vi "Prepare_dataST.vi"(1 "Active Sensors":bool[](array[boolean]), 2 "ranges":bool[](array[boolean]), 3 "Controls[]":refnum<vi>[](array[refnum]), 4 "Flag_215":bool, 5 "error in":errorcluster, 6 "struct":bool, 7 "chkeach_ch":bool) -> (12 "Meas_rang":i32[](array[numeric]), 13 "Refdata_struct":refnum<k24>[](array[refnum]), 15 "Meas_monitor_struct":refnum<k24>[](array[refnum]), 16 "Data_struct":refnum<k24>[](array[refnum]), 17 "Ref_monitordata_struct":refnum<k24>[](array[refnum]), 18 "Mergedata_struct":refnum<k24>[](array[refnum]), 19 "error out":errorcluster)   [LabVIEW 2017]
doc: "prepare data struct & hold instrument condition"
uses:
  D:/test/ILSTS/LV_IL/LV_IL_Sample_x64/DLL/STSProcess.dll
  DLL/STSProcess.dll
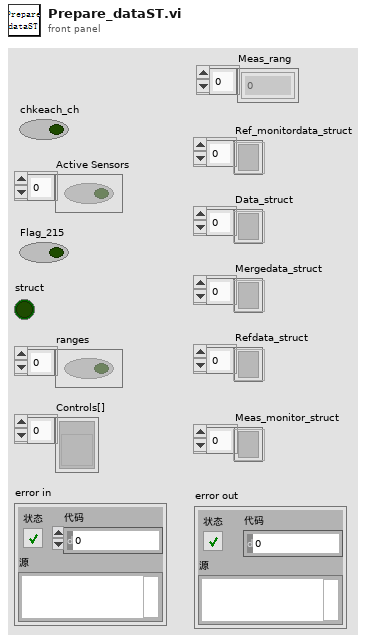
[diagram p1: front panel]
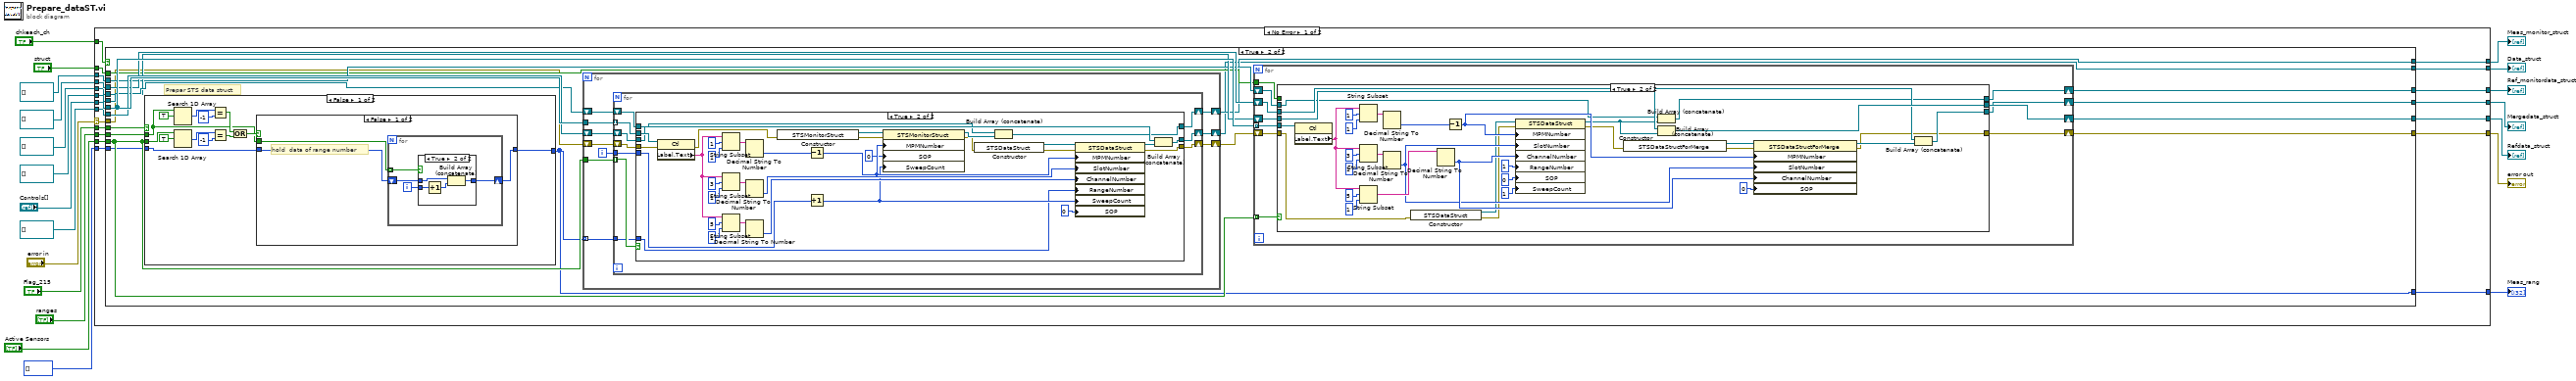
[diagram p0: block diagram]
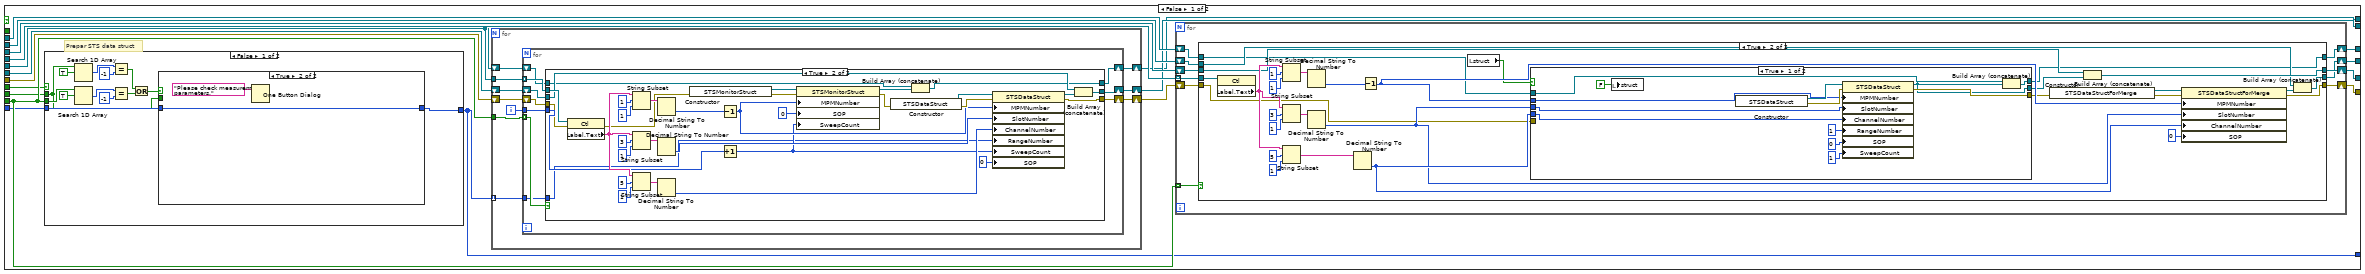
[diagram p2: hidden frame]
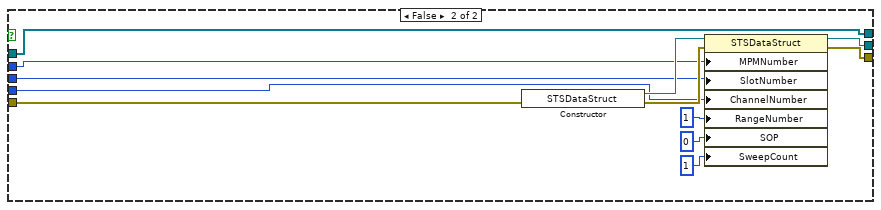
[diagram p4: hidden frame]
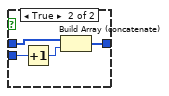
[diagram p7: hidden frame]
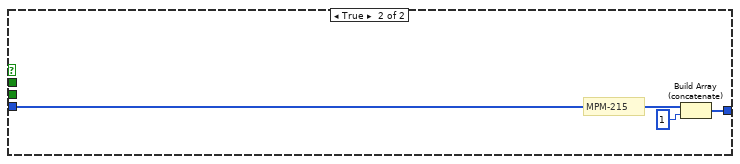
[diagram p8: hidden frame]
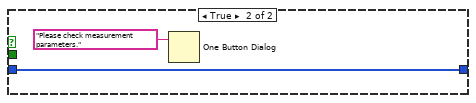
[diagram p12: hidden frame]
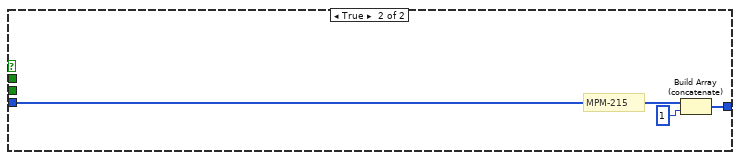
[diagram p13: hidden frame]
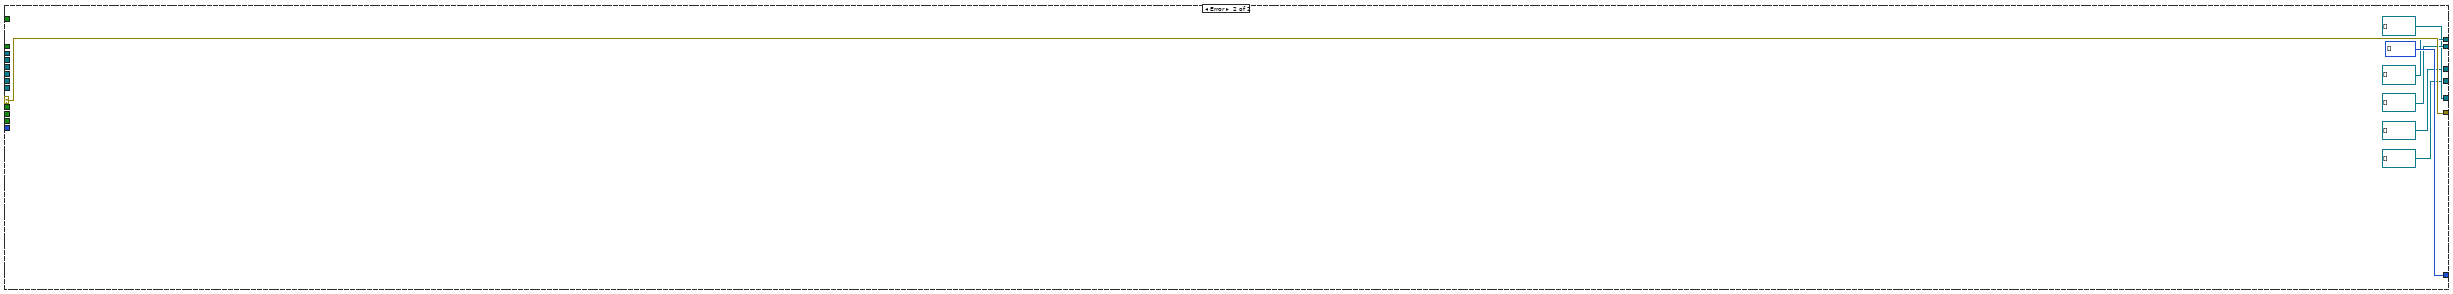
[diagram p14: hidden frame]
diagram:
  n1 = case shown="No Error" "error in" {
    selector: "error in" -> [w21 w378]
    tunnel: "ranges" -> [w40 _]
    tunnel: "Flag_215" -> [w39 _]
    tunnel: "Controls[]" -> [w38 _]
    tunnel: "Active Sensors" -> [w37 _]
    tunnel: "chkeach_ch" -> [w36 _]
    tunnel: "struct" -> [w35 _]
    tunnel: refnum<k24>[] [] ("Data_struct") -> [w34 _]
    tunnel: refnum<k24>[] [] ("Ref_monitordata_struct") -> [w33 _]
    tunnel: refnum<k24>[] [] ("Mergedata_struct") -> [w32 _]
    tunnel: refnum<k24>[] [] ("Meas_monitor_struct") -> [w31 _]
    tunnel: refnum<k24>[] [] ("Refdata_struct") -> [w30 _]
    tunnel: [w29 refnum<k24>[] [] ("Mergedata_struct")] -> w9
    tunnel: [w28 refnum<k24>[] [] ("Data_struct")] -> w8
    tunnel: [w27 refnum<k24>[] [] ("Meas_monitor_struct")] -> w7
    tunnel: [w26 refnum<k24>[] [] ("Refdata_struct")] -> w6
    tunnel: [w25 refnum<k24>[] [] ("Ref_monitordata_struct")] -> w5
    tunnel: i32[] [] ("Meas_rang") -> [w24 _]
    tunnel: [w23 i32[] [] ("Meas_rang")] -> w3
    tunnel: [w22 w378] -> w1
    frame No Error {
      n2 = case shown="True" w36 {
        tunnel: w37 -> [w58 w234]
        tunnel: w38 -> [w59 w235]
        tunnel: w34 -> [w57 w233]
        tunnel: w31 -> [w56 w232]
        tunnel: w30 -> [w55 w231]
        tunnel: w32 -> [w54 w230]
        tunnel: w33 -> [w53 w229]
        tunnel: w24 -> [w52 w228]
        tunnel: w39 -> [w51 w227]
        tunnel: w40 -> [w50 w226]
        tunnel: w35 -> [_ w225]
        tunnel: [w49 w222] -> w29
        tunnel: [w48 w223] -> w28
        tunnel: [w47 w224] -> w27
        tunnel: [w46 w220] -> w26
        tunnel: [w45 w221] -> w25
        tunnel: [w44 w219] -> w23
        tunnel: [w41 w218] -> w22
        tunnel: w21 -> [w42 w216]
        frame False {
          # "Prepar STS data struct"
          n3 = case shown="False" w51 {
            tunnel: w52 -> [w188 w215]
            tunnel: [w187 w213] -> w44
            tunnel: w58 -> [w198 _]
            tunnel: w50 -> [w186 _]
            frame False {
              n4 = Search 1D Array(1D array=w186, element=TRUE ("元素")) -> (index of element=w193:i32)  [unwired: 1 in]
              n5 = Search 1D Array(1D array=w198, element=TRUE ("元素")) -> (index of element=w196:i32)  [unwired: 1 in]
              n6 = Equal?(x=w193, y=-1) -> (x = y?=w191:bool)
              n7 = Equal?(x=w196, y=-1) -> (x = y?=w190:bool)
              n8 = Or(x=w191, y=w190) -> (x .or. y?=w189:bool)
              n9 = case shown="True" w189 {
                tunnel: w186 -> [w201 _]
                tunnel: w188 -> [w200 w211]
                tunnel: [w199 w211] -> w187
                frame False {
                  # "hold  data of range number"
                  n10 = for {
                    tunnel: w201 -> [w205] mode=indexing
                    shift-right: [w202] -> w199
                    shift-left: w200 -> [w204]
                    i -> [w203]
                    n11 = case shown="False" w205 {
                      tunnel: w204 -> [w206 w210]
                      tunnel: w203 -> [_ w208]
                      tunnel: [w206 w207] -> w202
                      frame False {
                      }
                      frame True {
                        n12 = Increment(x=w208) -> (x+1=w209:i32)
                        n13 = Build Array (concatenate)(w210, w209) -> (w207:i32[])
                      }
                    }
                  }
                }
                frame True {
                  n14 = One Button Dialog(message="Please check measurement parameters." ("消息")) -> ()  [unwired: 1 in, 1 out]
                }
              }
            }
            frame True {
              # "MPM-215"
              n15 = Build Array (concatenate)(w215, 1) -> (w213:i32[])
            }
          }
          n16 = for {
            tunnel: w58 -> [w138]
            tunnel: w59 -> [w137]
            tunnel: w44 -> [w136] mode=indexing
            shift-right: [w134] -> w48
            shift-left: w57 -> [w135]
            shift-right: [w131] -> w47
            shift-left: w56 -> [w132]
            shift-right: [w130] -> w43
            shift-left: w42 -> [w129]
            i -> [w133]
            n17 = for {
              tunnel: w138 -> [w148] mode=indexing
              tunnel: w137 -> [w147] mode=indexing
              tunnel: w136 -> [w139]
              shift-right: [w145] -> w134
              shift-left: w135 -> [w146]
              tunnel: w133 -> [w144]
              shift-right: [w142] -> w131
              shift-left: w132 -> [w143]
              shift-right: [w141] -> w130
              shift-left: w129 -> [w140]
              n18 = case shown="True" w148 {
                tunnel: w147 -> [_ w185]
                tunnel: w146 -> [w151 w171]
                tunnel: [w151 w169] -> w145
                tunnel: w144 -> [_ w166]
                tunnel: w143 -> [w150 w159]
                tunnel: [w150 w157] -> w142
                tunnel: [w149 w154] -> w141
                tunnel: w140 -> [w149 w153]
                tunnel: w139 -> [_ w152]
                frame False {
                }
                frame True {
                  n19 = property class="Ctl"(reference=w185, error in=w153) -> (error out=w156:errorcluster, "Label.Text"=w180:string)  [unwired: 1 out]
                  n20 = String Subset(string=w180, offset (0)=1 ("偏移量(0)"), length (rest)=1 ("长度（剩余）")) -> (substring=w176:string)
                  n21 = String Subset(string=w180, offset (0)=3 ("偏移量(0)"), length (rest)=1 ("长度（剩余）")) -> (substring=w177:string)
                  n22 = String Subset(string=w180, offset (0)=5 ("偏移量(0)"), length (rest)=1 ("长度（剩余）")) -> (substring=w175:string)
                  n23 = Decimal String To Number(string=w176) -> (number=w174:i32)  [unwired: 2 in, 1 out]
                  n24 = Decimal String To Number(string=w177) -> (number=w168:i32)  [unwired: 2 in, 1 out]
                  n25 = Decimal String To Number(string=w175) -> (number=w167:i32)  [unwired: 2 in, 1 out]
                  n26 = constructor class="STSMonitorStruct"(error in=w156) -> (reference out=w163:refnum<k24>, error out=w164:errorcluster)  [unwired: 2 in, 1 out]
                  n27 = Decrement(x=w174) -> (x-1=w162:i32)
                  n28 = Increment(x=w166) -> (x+1=w160:i32)
                  n29 = property class="STSMonitorStruct"(reference=w163, error in=w164, "MPMNumber"=w162, "SOP"=0, "SweepCount"=w160) -> (reference out=w158:refnum<k24>, error out=w155:errorcluster)
                  n30 = constructor class="STSDataStruct"(error in=w155) -> (reference out=w173:refnum<k24>, error out=w172:errorcluster)  [unwired: 2 in, 1 out]
                  n31 = Build Array (concatenate)(w159, w158) -> (w157:refnum<k24>[])
                  n32 = property on="属性节点" class="STSDataStruct"(reference=w173, error in=w172, "MPMNumber"=w162, "SlotNumber"=w168, "ChannelNumber"=w167, "RangeNumber"=w152, "SweepCount"=w160, "SOP"=0) -> (reference out=w170:refnum<k24>, error out=w154:errorcluster)
                  n33 = Build Array (concatenate)(w171, w170) -> (w169:refnum<k24>[])
                }
              }
            }
          }
          n34 = for {
            tunnel: w59 -> [w68] mode=indexing
            tunnel: w58 -> [w69] mode=indexing
            shift-right: [w66] -> w46
            shift-left: w55 -> [w67]
            shift-right: [w64] -> w49
            shift-left: w54 -> [w65]
            shift-right: [w62] -> w45
            shift-left: w53 -> [w63]
            shift-right: [w60] -> w41
            shift-left: w43 -> [w61]
            n35 = case shown="True" w69 {
              tunnel: w68 -> [_ w93]
              tunnel: w67 -> [w72 w84]
              tunnel: [w72 w82] -> w66
              tunnel: w65 -> [w73 w81]
              tunnel: [w73 w79] -> w64
              tunnel: w63 -> [w71 w78]
              tunnel: [w71 w77] -> w62
              tunnel: w61 -> [w70 w76]
              tunnel: [w70 w75] -> w60
              frame False {
              }
              frame True {
                n36 = property class="Ctl"(reference=w93) -> ("Label.Text"=w92:string)  [unwired: 1 in, 2 out]
                n37 = String Subset(string=w92, offset (0)=1 ("偏移量(0)"), length (rest)=1 ("长度（剩余）")) -> (substring=w96:string)
                n38 = String Subset(string=w92, offset (0)=3 ("偏移量(0)"), length (rest)=1 ("长度（剩余）")) -> (substring=w97:string)
                n39 = String Subset(string=w92, offset (0)=5 ("偏移量(0)"), length (rest)=1 ("长度（剩余）")) -> (substring=w95:string)
                n40 = Decimal String To Number(string=w96) -> (number=w94:i32)  [unwired: 2 in, 1 out]
                n41 = Decimal String To Number(string=w97) -> (number=w87:i32)  [unwired: 2 in, 1 out]
                n42 = Decimal String To Number(string=w95) -> (number=w88:i32)  [unwired: 2 in, 1 out]
                n43 = Decrement(x=w94) -> (x-1=w86:i32)
                n44 = local read "struct"() -> (w74:bool)
                n45 = case shown="True" w74 {
                  tunnel: w88 -> [w111 w123]
                  tunnel: w87 -> [w110 w122]
                  tunnel: w86 -> [w109 w121]
                  tunnel: [w108 w120] -> w85
                  tunnel: [w106 w119] -> w83
                  tunnel: w78 -> [w107 w118]
                  tunnel: [w105 w118] -> w77
                  tunnel: w76 -> [_ w117]
                  frame True {
                    n46 = local write "struct"(FALSE ("struct")) -> ()
                    n47 = constructor class="STSDataStruct"() -> (reference out=w115:refnum<k24>, error out=w116:errorcluster)  [unwired: 3 in, 1 out]
                    n48 = property class="STSDataStruct"(reference=w115, error in=w116, "MPMNumber"=w109, "SlotNumber"=w110, "ChannelNumber"=w111, "RangeNumber"=1, "SOP"=0, "SweepCount"=1) -> (reference out=w106:refnum<k24>, error out=w108:errorcluster)
                    n49 = Build Array (concatenate)(w107, w106) -> (w105:refnum<k24>[])
                  }
                  frame False {
                    n50 = constructor class="STSDataStruct"(error in=w117) -> (reference out=w127:refnum<k24>, error out=w128:errorcluster)  [unwired: 2 in, 1 out]
                    n51 = property class="STSDataStruct"(reference=w127, error in=w128, "MPMNumber"=w121, "SlotNumber"=w122, "ChannelNumber"=w123, "RangeNumber"=1, "SOP"=0, "SweepCount"=1) -> (reference out=w119:refnum<k24>, error out=w120:errorcluster)
                  }
                }
                n52 = constructor class="STSDataStructForMerge"(error in=w85) -> (reference out=w91:refnum<k24>, error out=w90:errorcluster)  [unwired: 2 in, 1 out]
                n53 = Build Array (concatenate)(w84, w83) -> (w82:refnum<k24>[])
                n54 = property class="STSDataStructForMerge"(reference=w91, error in=w90, "MPMNumber"=w86, "SlotNumber"=w87, "ChannelNumber"=w88, "SOP"=0) -> (reference out=w80:refnum<k24>, error out=w75:errorcluster)
                n55 = Build Array (concatenate)(w81, w80) -> (w79:refnum<k24>[])
              }
            }
          }
        }
        frame True {
          # "Prepar STS data struct"
          n56 = case shown="False" w227 {
            tunnel: w228 -> [w344 w371]
            tunnel: [w343 w369] -> w219
            tunnel: w234 -> [w354 _]
            tunnel: w226 -> [w342 _]
            frame False {
              n57 = Search 1D Array(1D array=w342, element=TRUE ("元素")) -> (index of element=w349:i32)  [unwired: 1 in]
              n58 = Search 1D Array(1D array=w354, element=TRUE ("元素")) -> (index of element=w352:i32)  [unwired: 1 in]
              n59 = Equal?(x=w349, y=-1) -> (x = y?=w347:bool)
              n60 = Equal?(x=w352, y=-1) -> (x = y?=w346:bool)
              n61 = Or(x=w347, y=w346) -> (x .or. y?=w345:bool)
              n62 = case shown="False" w345 {
                tunnel: w342 -> [w357 _]
                tunnel: w344 -> [w356 w367]
                tunnel: [w355 w367] -> w343
                frame False {
                  # "hold  data of range number"
                  n63 = for {
                    tunnel: w357 -> [w361] mode=indexing
                    shift-right: [w358] -> w355
                    shift-left: w356 -> [w360]
                    i -> [w359]
                    n64 = case shown="True" w361 {
                      tunnel: w360 -> [w362 w366]
                      tunnel: w359 -> [_ w364]
                      tunnel: [w362 w363] -> w358
                      frame False {
                      }
                      frame True {
                        n65 = Increment(x=w364) -> (x+1=w365:i32)
                        n66 = Build Array (concatenate)(w366, w365) -> (w363:i32[])
                      }
                    }
                  }
                }
                frame True {
                  n67 = One Button Dialog(message="Please check measurement parameters." ("消息")) -> ()  [unwired: 1 in, 1 out]
                }
              }
            }
            frame True {
              # "MPM-215"
              n68 = Build Array (concatenate)(w371, 1) -> (w369:i32[])
            }
          }
          n69 = for {
            tunnel: w234 -> [w294]
            tunnel: w235 -> [w293]
            tunnel: w219 -> [w292] mode=indexing
            shift-right: [w290] -> w223
            shift-left: w233 -> [w291]
            shift-right: [w287] -> w224
            shift-left: w232 -> [w288]
            shift-right: [w286] -> w217
            shift-left: w216 -> [w285]
            i -> [w289]
            n70 = for {
              tunnel: w294 -> [w304] mode=indexing
              tunnel: w293 -> [w303] mode=indexing
              tunnel: w292 -> [w295]
              shift-right: [w301] -> w290
              shift-left: w291 -> [w302]
              tunnel: w289 -> [w300]
              shift-right: [w298] -> w287
              shift-left: w288 -> [w299]
              shift-right: [w297] -> w286
              shift-left: w285 -> [w296]
              n71 = case shown="True" w304 {
                tunnel: w303 -> [_ w341]
                tunnel: w302 -> [w307 w327]
                tunnel: [w307 w325] -> w301
                tunnel: w300 -> [_ w322]
                tunnel: w299 -> [w306 w315]
                tunnel: [w306 w313] -> w298
                tunnel: [w305 w310] -> w297
                tunnel: w296 -> [w305 w309]
                tunnel: w295 -> [_ w308]
                frame False {
                }
                frame True {
                  n72 = property class="Ctl"(reference=w341, error in=w309) -> (error out=w311:errorcluster, "Label.Text"=w336:string)  [unwired: 1 out]
                  n73 = String Subset(string=w336, offset (0)=1 ("偏移量(0)"), length (rest)=1 ("长度（剩余）")) -> (substring=w332:string)
                  n74 = String Subset(string=w336, offset (0)=3 ("偏移量(0)"), length (rest)=1 ("长度（剩余）")) -> (substring=w333:string)
                  n75 = String Subset(string=w336, offset (0)=5 ("偏移量(0)"), length (rest)=1 ("长度（剩余）")) -> (substring=w331:string)
                  n76 = Decimal String To Number(string=w332) -> (number=w330:i32)  [unwired: 2 in, 1 out]
                  n77 = Decimal String To Number(string=w333) -> (number=w324:i32)  [unwired: 2 in, 1 out]
                  n78 = Decimal String To Number(string=w331) -> (number=w323:i32)  [unwired: 2 in, 1 out]
                  n79 = constructor class="STSMonitorStruct"(error in=w311) -> (reference out=w319:refnum<k24>, error out=w320:errorcluster)  [unwired: 2 in, 1 out]
                  n80 = Decrement(x=w330) -> (x-1=w318:i32)
                  n81 = Increment(x=w322) -> (x+1=w316:i32)
                  n82 = property class="STSMonitorStruct"(reference=w319, error in=w320, "MPMNumber"=w318, "SOP"=0, "SweepCount"=w316) -> (reference out=w314:refnum<k24>, error out=w312:errorcluster)
                  n83 = constructor class="STSDataStruct"(error in=w312) -> (reference out=w329:refnum<k24>, error out=w328:errorcluster)  [unwired: 2 in, 1 out]
                  n84 = Build Array (concatenate)(w315, w314) -> (w313:refnum<k24>[])
                  n85 = property on="属性节点" class="STSDataStruct"(reference=w329, error in=w328, "MPMNumber"=w318, "SlotNumber"=w324, "ChannelNumber"=w323, "RangeNumber"=w308, "SweepCount"=w316, "SOP"=0) -> (reference out=w326:refnum<k24>, error out=w310:errorcluster)
                  n86 = Build Array (concatenate)(w327, w326) -> (w325:refnum<k24>[])
                }
              }
            }
          }
          n87 = for {
            tunnel: w235 -> [w245] mode=indexing
            tunnel: w234 -> [w246] mode=indexing
            shift-right: [w243] -> w220
            shift-left: w231 -> [w244]
            shift-right: [w241] -> w222
            shift-left: w230 -> [w242]
            shift-right: [w239] -> w221
            shift-left: w229 -> [w240]
            tunnel: w225 -> [w238]
            shift-right: [w237] -> w218
            shift-left: w217 -> [w236]
            n88 = case shown="True" w246 {
              tunnel: w245 -> [_ w274]
              tunnel: w244 -> [w249 w265]
              tunnel: [w249 w263] -> w243
              tunnel: w242 -> [w250 w262]
              tunnel: [w250 w260] -> w241
              tunnel: w240 -> [w248 w259]
              tunnel: [w248 w258] -> w239
              tunnel: w238 -> [_ _]
              tunnel: [w247 w257] -> w237
              tunnel: w236 -> [w247 w251]
              frame False {
              }
              frame True {
                n89 = property class="Ctl"(reference=w274) -> ("Label.Text"=w273:string)  [unwired: 1 in, 2 out]
                n90 = String Subset(string=w273, offset (0)=1 ("偏移量(0)"), length (rest)=1 ("长度（剩余）")) -> (substring=w277:string)
                n91 = String Subset(string=w273, offset (0)=3 ("偏移量(0)"), length (rest)=1 ("长度（剩余）")) -> (substring=w278:string)
                n92 = String Subset(string=w273, offset (0)=5 ("偏移量(0)"), length (rest)=1 ("长度（剩余）")) -> (substring=w276:string)
                n93 = Decimal String To Number(string=w277) -> (number=w275:i32)  [unwired: 2 in, 1 out]
                n94 = Decimal String To Number(string=w278) -> (number=w268:i32)  [unwired: 2 in, 1 out]
                n95 = constructor class="STSDataStruct"(error in=w251) -> (reference out=w255:refnum<k24>, error out=w256:errorcluster)  [unwired: 2 in, 1 out]
                n96 = Decimal String To Number(string=w276) -> (number=w269:i32)  [unwired: 2 in, 1 out]
                n97 = Decrement(x=w275) -> (x-1=w267:i32)
                n98 = property class="STSDataStruct"(reference=w255, error in=w256, "MPMNumber"=w267, "SlotNumber"=w268, "ChannelNumber"=w269, "RangeNumber"=1, "SOP"=0, "SweepCount"=1) -> (reference out=w264:refnum<k24>, error out=w266:errorcluster)
                n99 = constructor class="STSDataStructForMerge"(error in=w266) -> (reference out=w272:refnum<k24>, error out=w271:errorcluster)  [unwired: 2 in, 1 out]
                n100 = Build Array (concatenate)(w259, w264) -> (w258:refnum<k24>[])
                n101 = Build Array (concatenate)(w265, w264) -> (w263:refnum<k24>[])
                n102 = property class="STSDataStructForMerge"(reference=w272, error in=w271, "MPMNumber"=w267, "SlotNumber"=w268, "ChannelNumber"=w269, "SOP"=0) -> (reference out=w261:refnum<k24>, error out=w257:errorcluster)
                n103 = Build Array (concatenate)(w262, w261) -> (w260:refnum<k24>[])
              }
            }
          }
        }
      }
    }
    frame Error {
    }
  }
  "Ref_monitordata_struct" <- w5
  "Mergedata_struct" <- w9
  "Refdata_struct" <- w6
  "Meas_monitor_struct" <- w7
  "Data_struct" <- w8
  "Meas_rang" <- w3
  "error out" <- w1
